vi "loginProgram.vi"() -> ()   [LabVIEW 2014]
panel:
  out "提示":string
  in  "退出 2":bool
  in  "登录 2":bool
  in  "密码":string
  in  "用户名":string
  out "错误输出":errorcluster
  in  "错误输入（无错误）":errorcluster
  out "password":string
  out "username":string
  # "低压元器件应用验证测试系统"
  # "用户登录"
  # "用户名"
  # "密码"
  # "陕西嘉年盛达电子科技有限公司\n版本：V1.0"
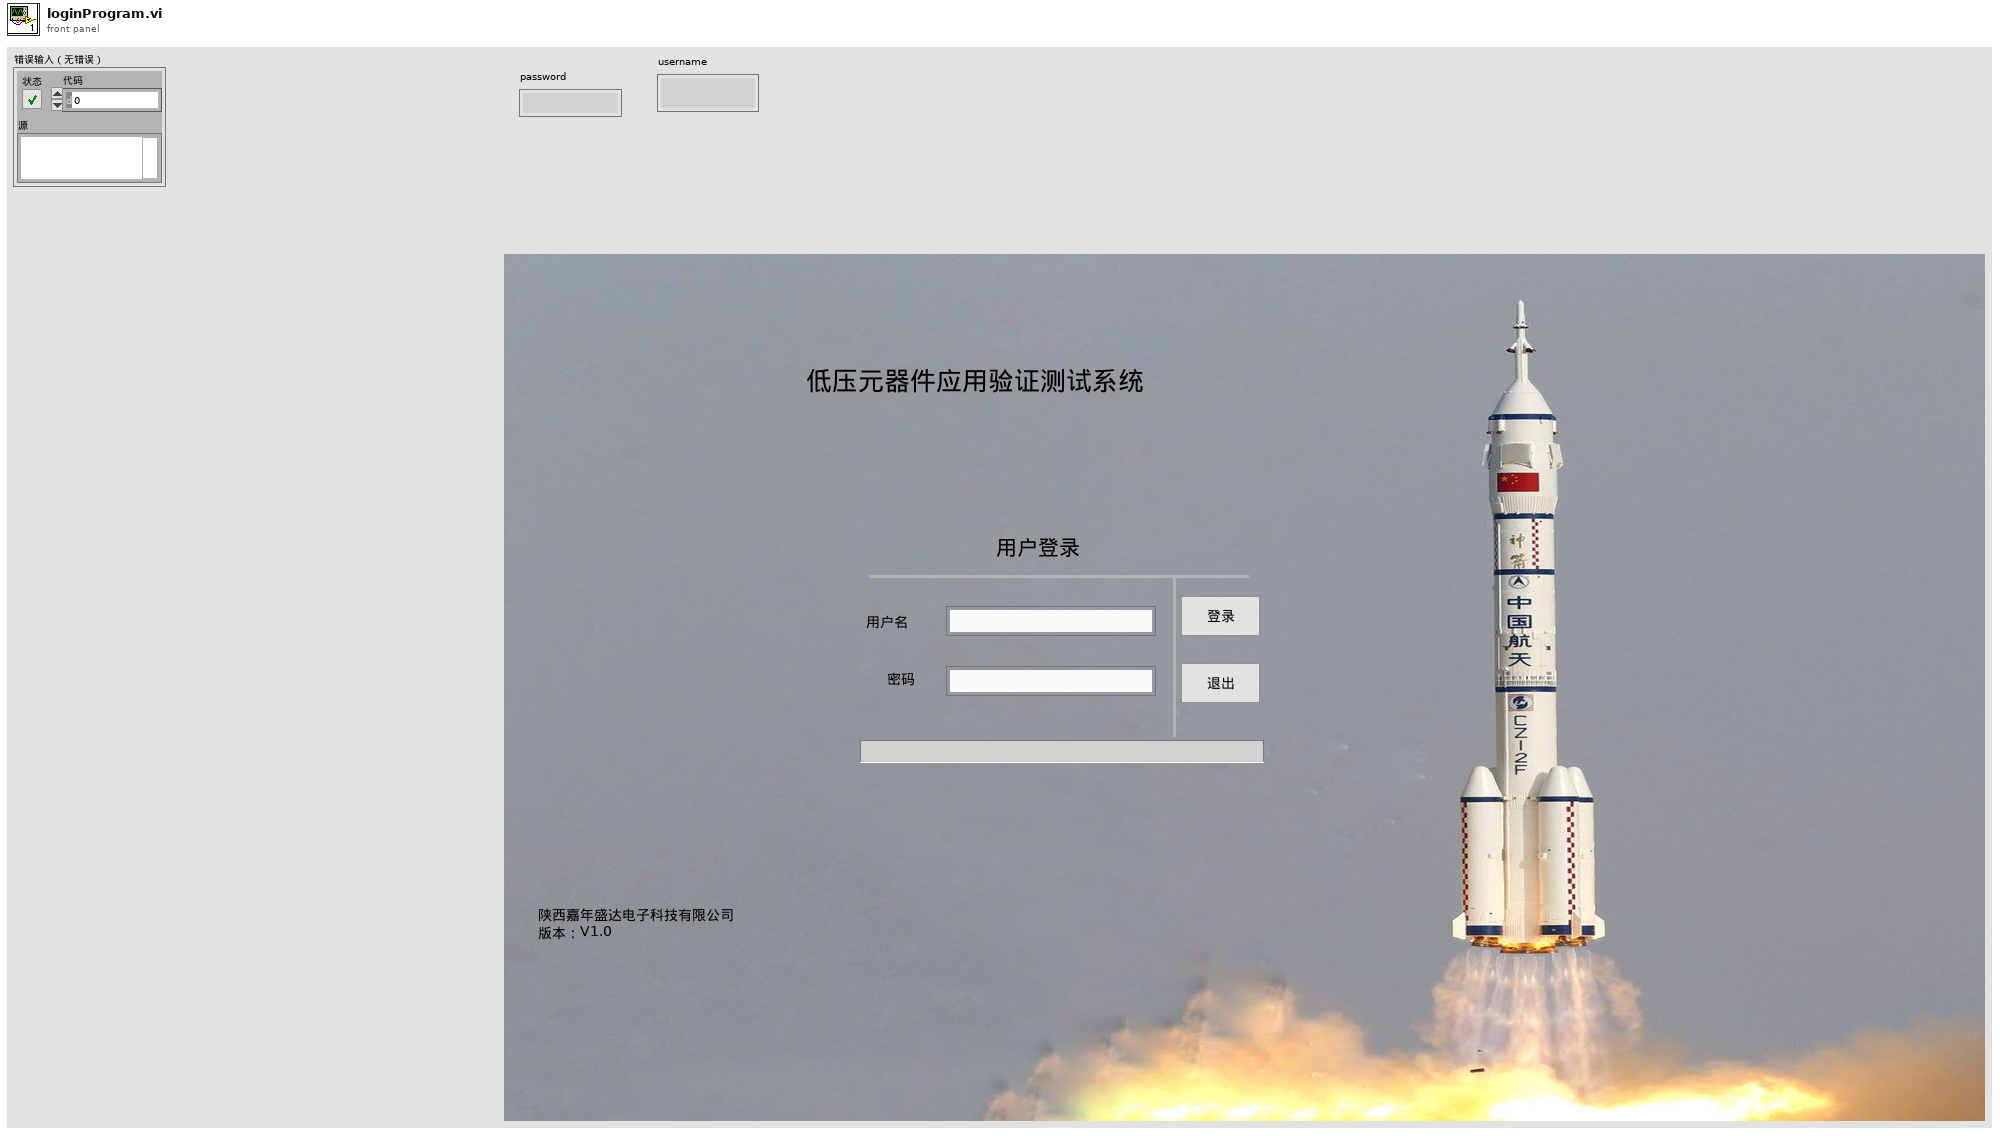
[diagram p1: front panel]
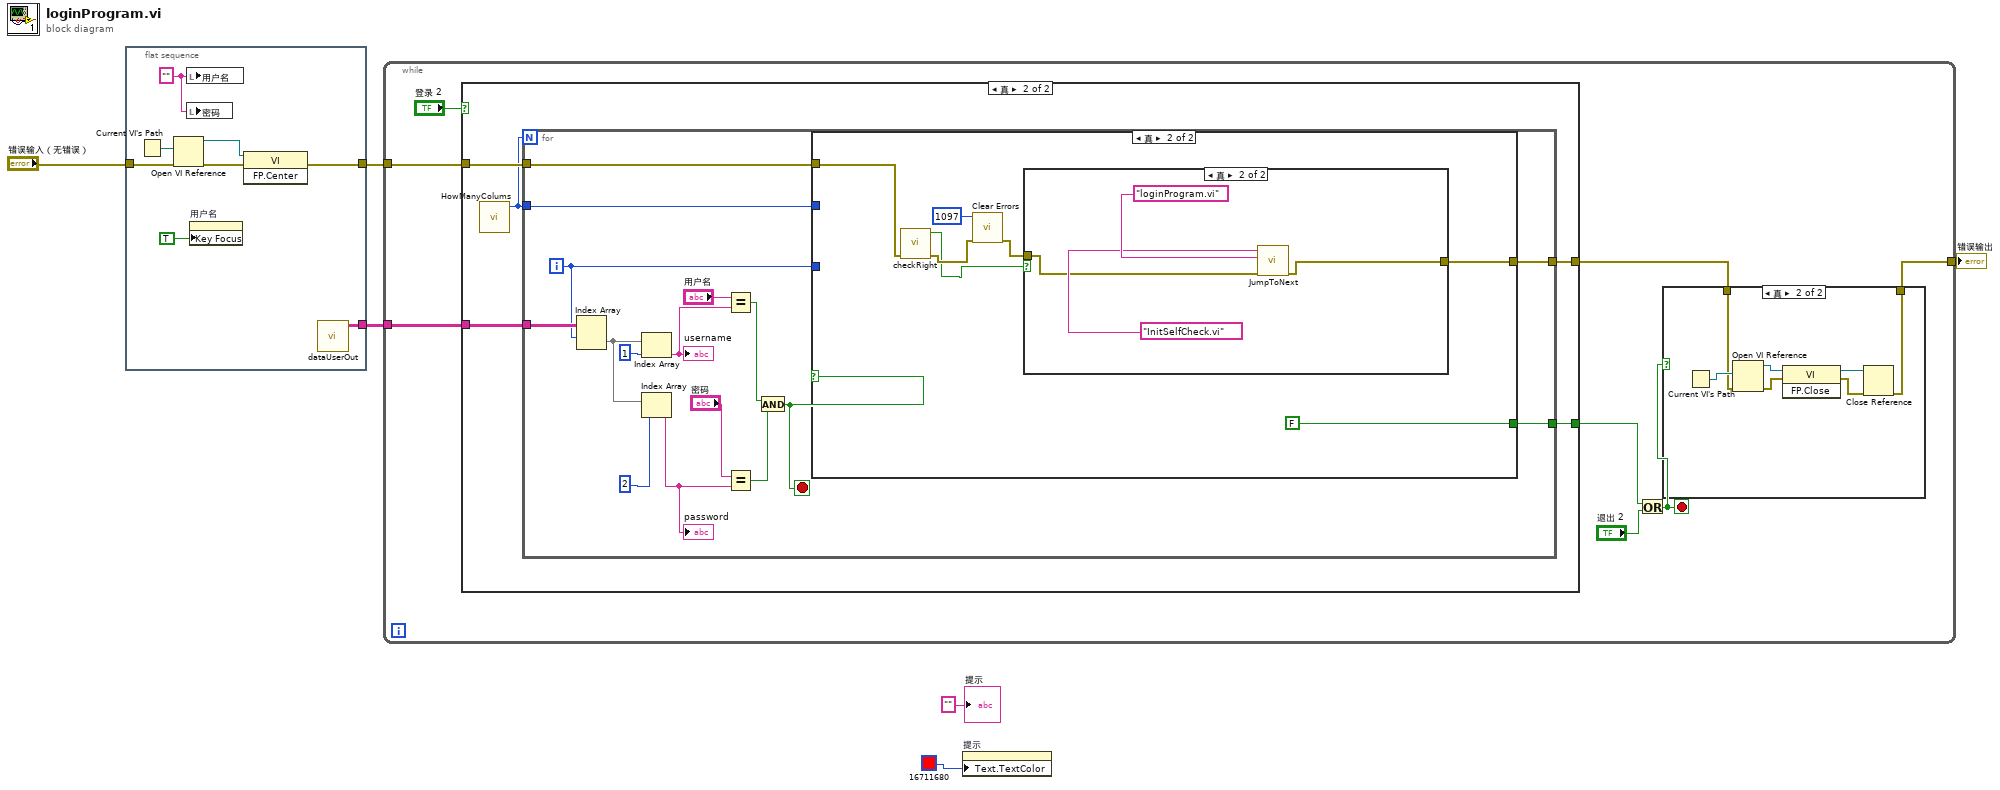
[diagram p0: block diagram]
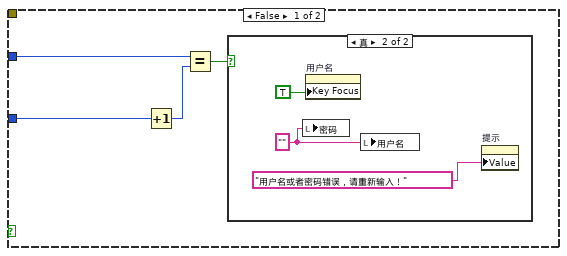
[diagram p4: hidden frame]
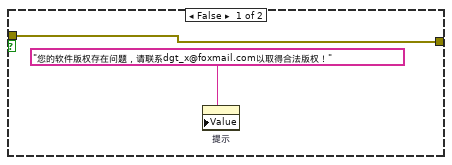
[diagram p6: hidden frame]
diagram:
  n1 = flat-sequence {
    tunnel: [w14] -> w6
    tunnel: "错误输入（无错误）" -> [w10]
    tunnel: [w8] -> w4
    frame #0 {
      w11 = ""
      n2 = Current VI's Path() -> (path=w12:path)
      n3 = Open VI Reference(vi path=w12, error in (no error)=w10) -> (vi reference=w13:refnum<vi>, error out=w9:errorcluster)  [unwired: 4 in]
      n4 = local write "用户名"(w11) -> ()
      n5 = local write "密码"(w11) -> ()
      n6 = property on="用户名" class="Str"("Key Focus"=TRUE ("键选中")) -> ()  [unwired: 2 in, 2 out]
      n7 = invoke class="VI" method="FP.Center"(reference=w13, error in=w9) -> (error out=w8:errorcluster)  [unwired: 1 in, 2 out]
      n8 = call "dataUserOut.vi"() -> ("Data"=w14:string[][])  [unwired: 10 in, 1 out]
    }
  }
  n9 = while {
    tunnel: w6 -> [w22]
    tunnel: w4 -> [w21]
    tunnel: [w15] -> w3
    stop <- w17 stop-if-true
    n10 = case shown="真" "登录 2" {
      tunnel: w22 -> [_ w34]
      tunnel: w21 -> [_ w35]
      tunnel: [_ w32] -> w16
      tunnel: [_ w31] -> w18
      frame False {
      }
      frame True {
        n11 = call "HowManyColums.vi"() -> ("数目"=w33:i32)  [unwired: 10 in, 1 out]
        n12 = for {
          N: w33 -> [_]
          tunnel: w35 -> [w38]
          tunnel: w34 -> [w42]
          tunnel: w33 -> [w40]
          tunnel: [w37] -> w32
          tunnel: [w36] -> w31
          i -> [w41]
          stop <- w39 stop-if-true
          n13 = Index Array(array=w42, index (row)=w41) -> (element=w51:string[])  [unwired: 1 in]
          n14 = Index Array(array=w51, index=1 ("索引 (行)")) -> (element=w48:string)
          "username" <- w48
          n15 = Index Array(array=w51, index=2 ("索引 (行)")) -> (element=w46:string)
          "password" <- w46
          n16 = Equal?(x="用户名", y=w48) -> (x = y?=w47:bool)
          n17 = Equal?(x="密码", y=w46) -> (x = y?=w45:bool)
          n18 = And(x=w47, y=w45) -> (x .and. y?=w39:bool)
          n19 = case shown="真" w39 {
            tunnel: w41 -> [w55 _]
            tunnel: w40 -> [w52 _]
            tunnel: w38 -> [_ w63]
            tunnel: [_ w65] -> w37
            tunnel: [_ FALSE] -> w36
            frame False {
              n20 = Increment(x=w55) -> (x+1=w54:i32)
              n21 = Equal?(x=w52, y=w54) -> (x = y?=w53:bool)
              n22 = case shown="真" w53 {
                frame False {
                }
                frame True {
                  w57 = ""
                  n23 = local write "密码"(w57) -> ()
                  n24 = property on="用户名" class="Str"("Key Focus"=TRUE ("键选中")) -> ()  [unwired: 2 in, 2 out]
                  n25 = local write "用户名"(w57) -> ()
                  n26 = property on="提示" class="Str"("Value"="用户名或者密码错误，请重新输入！" ("消息")) -> ()  [unwired: 2 in, 2 out]
                }
              }
            }
            frame True {
              n27 = call "checkRight.vi"("错误输入（无错误）"=w63) -> ("错误输出"=w62:errorcluster, "是否合法"=w59:bool)  [unwired: 9 in]
              n28 = call <vilib>:"Clear Errors.vi"("error in (no error)"=w62, "specific error code to clear (0: all)"=1097) -> ("error out"=w61:errorcluster)  [unwired: 4 in, 1 out]
              n29 = case shown="真" w59 {
                tunnel: [w67 w69] -> w65
                tunnel: w61 -> [w67 w68]
                frame False {
                  n30 = property on="提示" class="Str"("Value"="您的软件版权存在问题，请联系dgt_x@foxmail.com以取得合法版权！") -> ()  [unwired: 2 in, 2 out]
                }
                frame True {
                  n31 = call "JumpToNext.vi"("错误输入（无错误）"=w68, "要关闭的VI"="loginProgram.vi", "要打开的VI"="InitSelfCheck.vi") -> ("错误输出"=w69:errorcluster)  [unwired: 8 in]
                }
              }
            }
          }
        }
      }
    }
    n32 = Or(x=w18, y="退出 2") -> (x .or. y?=w17:bool)
    n33 = case shown="真" w17 {
      tunnel: w16 -> [w23 w25]
      tunnel: [w23 w24] -> w15
      frame False {
      }
      frame True {
        n34 = Current VI's Path() -> (path=w30:path)
        n35 = Open VI Reference(vi path=w30, error in (no error)=w25) -> (vi reference=w29:refnum<vi>, error out=w28:errorcluster)  [unwired: 4 in]
        n36 = invoke class="VI" method="FP.Close"(reference=w29, error in=w28) -> (reference out=w26:refnum<vi>, error out=w27:errorcluster)  [unwired: 1 in, 1 out]
        n37 = Close Reference(reference=w26, error in (no error)=w27) -> (error out=w24:errorcluster)
      }
    }
  }
  "错误输出" <- w3
  n38 = property on="提示" class="Str"("Text.TextColor"=u32 16711680) -> ()  [unwired: 2 in, 2 out]
  "提示" <- "" ("提示")
